vi "SetWindowMaximumSize.vi"(8 "No Error":errorcluster, 9 "h":i32, 10 "w":i32, 11 "Window [SDL_Window *]":i64 format="%.0x") -> (0 "Error Out":errorcluster)   [LabVIEW 2024, in "SDL3.lvlib" / "Video.lvlib"]
doc: "<B>Summary</B>\nSet the maximum size of a window's client area.\n\n<B>Thread Safety</B>\nThis function should only be called on the main thread."
uses:
  Video.lvlib
  <vilib>/Utility/error.llb/Error Cluster From Error Code.vi
  Error/Error.lvlib
  Lib/SDL3-32.dll
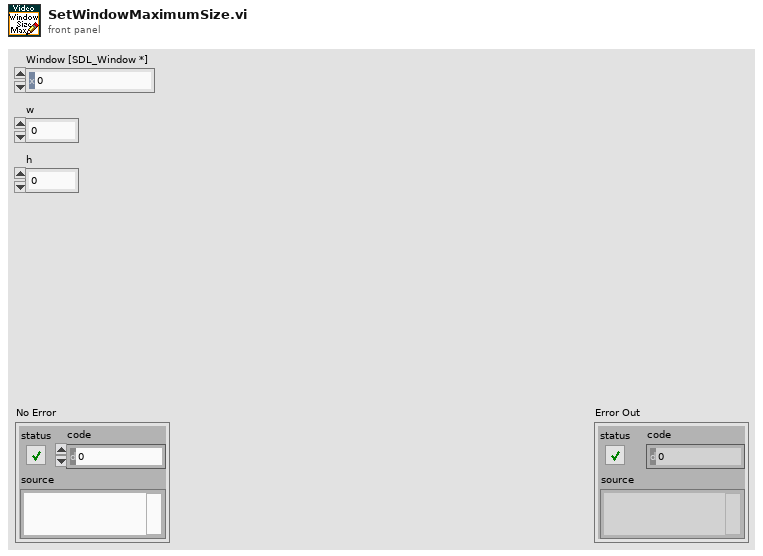
[diagram p1: front panel]
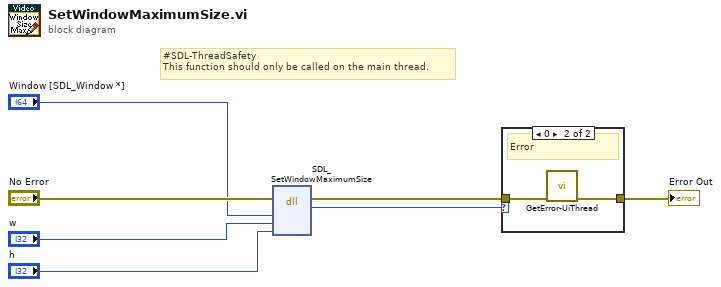
[diagram p0: block diagram]
diagram:
  # "#SDL-ThreadSafety\nThis function should only be called on the main thread."
  n1 = dll-call lib="C:/Users/Thomas/Documents/Projects/LV-SDL3/Lib/SDL3-*.*" fn="SDL_SetWindowMaximumSize"(error in="No Error", "window"="Window [SDL_Window *]", "w"="w", "h"="h") -> (error out=w2:errorcluster, "return type"=w1:i32)  [unwired: 5 in, 1 out]
  n2 = case shown="0" w1 {
    tunnel: w2 -> [w8 w10]
    tunnel: [w8 w9] -> w6
    frame Default {
      # "Ok"
    }
    frame 0 {
      # "Error"
      n3 = call "GetError-UiThread.vi"("No Error"=w10) -> ("error out"=w9:errorcluster)  [unwired: 10 in]
    }
  }
  "Error Out" <- w6
